vi "CirclesExample.vi"() -> (0 "XY Graph":cluster{dbl[], dbl[]}[](graph))   [LabVIEW 2014]
panel:
  in  "Array":T1(array[cluster])
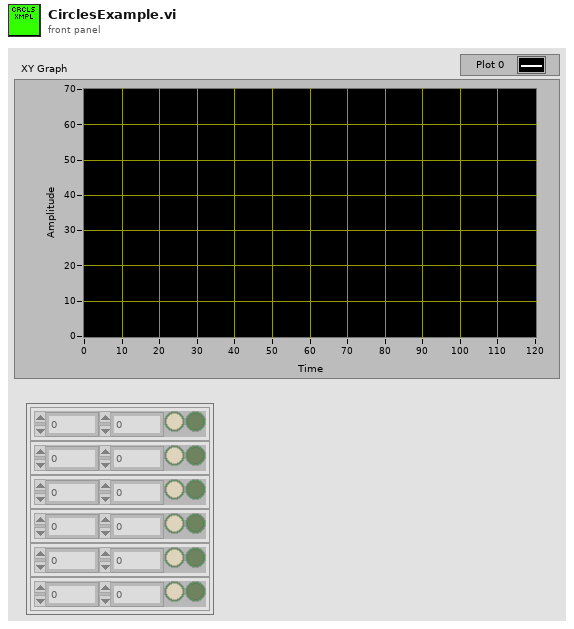
[diagram p1: front panel]
types:
  T1 = cluster{"y":dbl, "x":dbl, "Fout":bool, "Goed 2":bool}[]
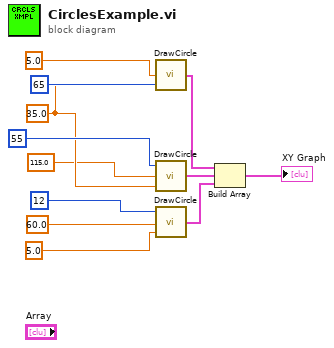
[diagram p0: block diagram]
diagram:
  w5 = 35.0 ("y")
  n1 = call "DrawCircle.vi"("y"=w5, "x"=5.0, "r"=65) -> ("XY Graph"=w10:cluster{dbl[], dbl[]})
  n2 = call "DrawCircle.vi"("y"=w5, "x"=115.0, "r"=55) -> ("XY Graph"=w11:cluster{dbl[], dbl[]})
  n3 = call "DrawCircle.vi"("y"=5.0, "x"=60.0, "r"=12) -> ("XY Graph"=w12:cluster{dbl[], dbl[]})
  n4 = Build Array "Build Array"(w10, w11, w12) -> (→"XY Graph":cluster{dbl[], dbl[]}[])
